vi "Callback Template.vi"(8 "error in (no error)":errorcluster, 9 "Scope":variant, 11 "Value":variant) -> (0 "error out":errorcluster)   [LabVIEW 2017]
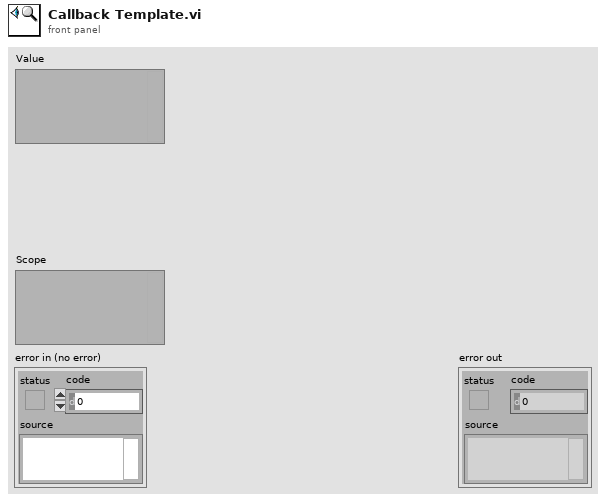
[diagram p1: front panel]
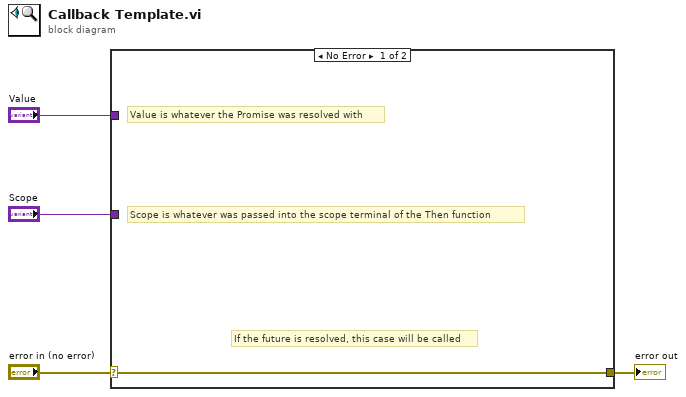
[diagram p0: block diagram]
diagram:
  n1 = case shown="No Error" "error in (no error)" {
    selector: "error in (no error)" -> [w5 w6]
    tunnel: [w5 w6] -> w3
    tunnel: "Scope" -> [_ _]
    tunnel: "Value" -> [_ _]
    frame No Error {
      # "Value is whatever the Promise was resolved with"
      # "Scope is whatever was passed into the scope terminal of the Then function"
      # "If the future is resolved, this case will be called"
    }
    frame Error {
      # "If the future is Rejected, this case will be called with the error in as the reason"
    }
  }
  "error out" <- w3
